vi "xorychannelchosen.vi"(1 "AO channels":u32) -> (0 "x .or. y?":bool)   [LabVIEW 2015]
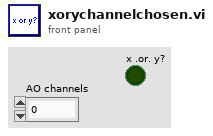
[diagram p1: front panel]
types:
  T1 = cluster{"StageS":i32, "StageL":i32, "currmeas data dir":path, "image OD":u16, "contour OD":u16, "point OD":u16, "AOlines":tag[], "AIlines":tag[], "CI lines":tag[], "DO lines":tag[], "AO names":string[], "CI names":string[], "AI names":string[], "DO names":string[], "CIextensions":string[], "AIextensions":string[], "Voltage to Ygalvo":i32, "Voltage to Xgalvo":i32, "Voltage to patch":i32, "640 shutter":i32, "2P shutter":i32, "LT timestamp":i32, "Vp":i32, "Ip":i32, "camera trigger":i32, "master data dir":path}
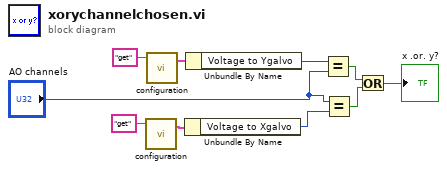
[diagram p0: block diagram]
diagram:
  n1 = call "configuration.vi"("command"="get") -> ("config out"=w8:T1)  [unwired: 2 in, 1 out]
  n2 = call "configuration.vi"("command"="get") -> ("config out"=w2:T1)  [unwired: 2 in, 1 out]
  n3 = Unbundle By Name(w8) -> ("Voltage to Xgalvo"=w5:i32)
  n4 = Unbundle By Name(w2) -> ("Voltage to Ygalvo"=w6:i32)
  n5 = Equal?(x=w6, y="AO channels") -> (x = y?=w9:bool)
  n6 = Equal?(x="AO channels", y=w5) -> (x = y?=w10:bool)
  n7 = Or(x=w9, y=w10) -> (x .or. y?=→"x .or. y?":bool)
